vi "U3 eDO Example.vi"() -> (0 "error out":errorcluster)   [LabVIEW 2021]
panel:
  in  "State":bool
  in  "Channel":i32=4
  in  "FirstFound":bool=TRUE
  in  "Address":string="1"
  out "Error Message":string
  # "Updates 1 digital output using the UD easy function eDO."
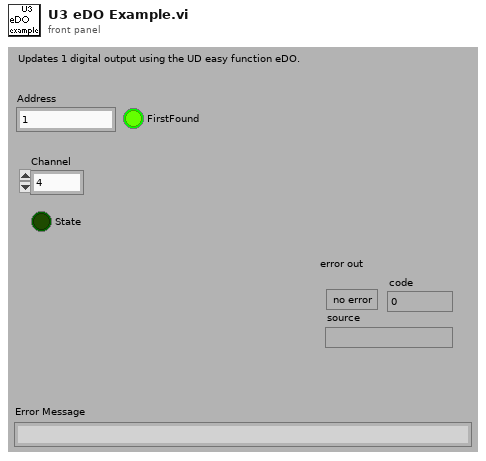
[diagram p1: front panel]
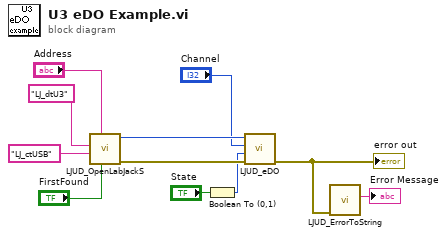
[diagram p0: block diagram]
diagram:
  n1 = call "LJUD_OpenLabJackS.vi"("FirstFound"="FirstFound", "Address"="Address", "ConnectionType"="LJ_ctUSB", "DeviceType"="LJ_dtU3") -> ("error out"=w5:errorcluster, "Handle"=w6:i32)  [unwired: 5 in, 1 out]
  n2 = Boolean To (0,1)(Boolean="State") -> (0, 1=w1:i16)
  n3 = call "LJUD_eDO.vi"("error in"=w5, "State"=w1, "Channel"="Channel", "Handle In"=w6) -> ("error out"=w4:errorcluster)  [unwired: 6 in, 1 out]
  "error out" <- w4
  n4 = call "LJUD_ErrorToString.vi"("error in"=w4) -> ("String"=→"Error Message":string)  [unwired: 10 in]
